vi "Get Selected Controls - List of properties.vi"(8 "error in (no error)":errorcluster, 10 "List of Properties":string[](array[string]), 11 "Data in":T2) -> (0 "error out":errorcluster, 3 "Selected Ctrls - List of Properties":T1)   [LabVIEW 2021, in "Control Property Tree.lvlib"]
uses:
  Control Property Tree.lvlib
  Module Data--cluster.ctl
  Ctrl Properties Map Data.ctl
  Property array.ctl
  Selected Ctrls - List of Controls.ctl
  Selected Ctrls - List of Properties.ctl
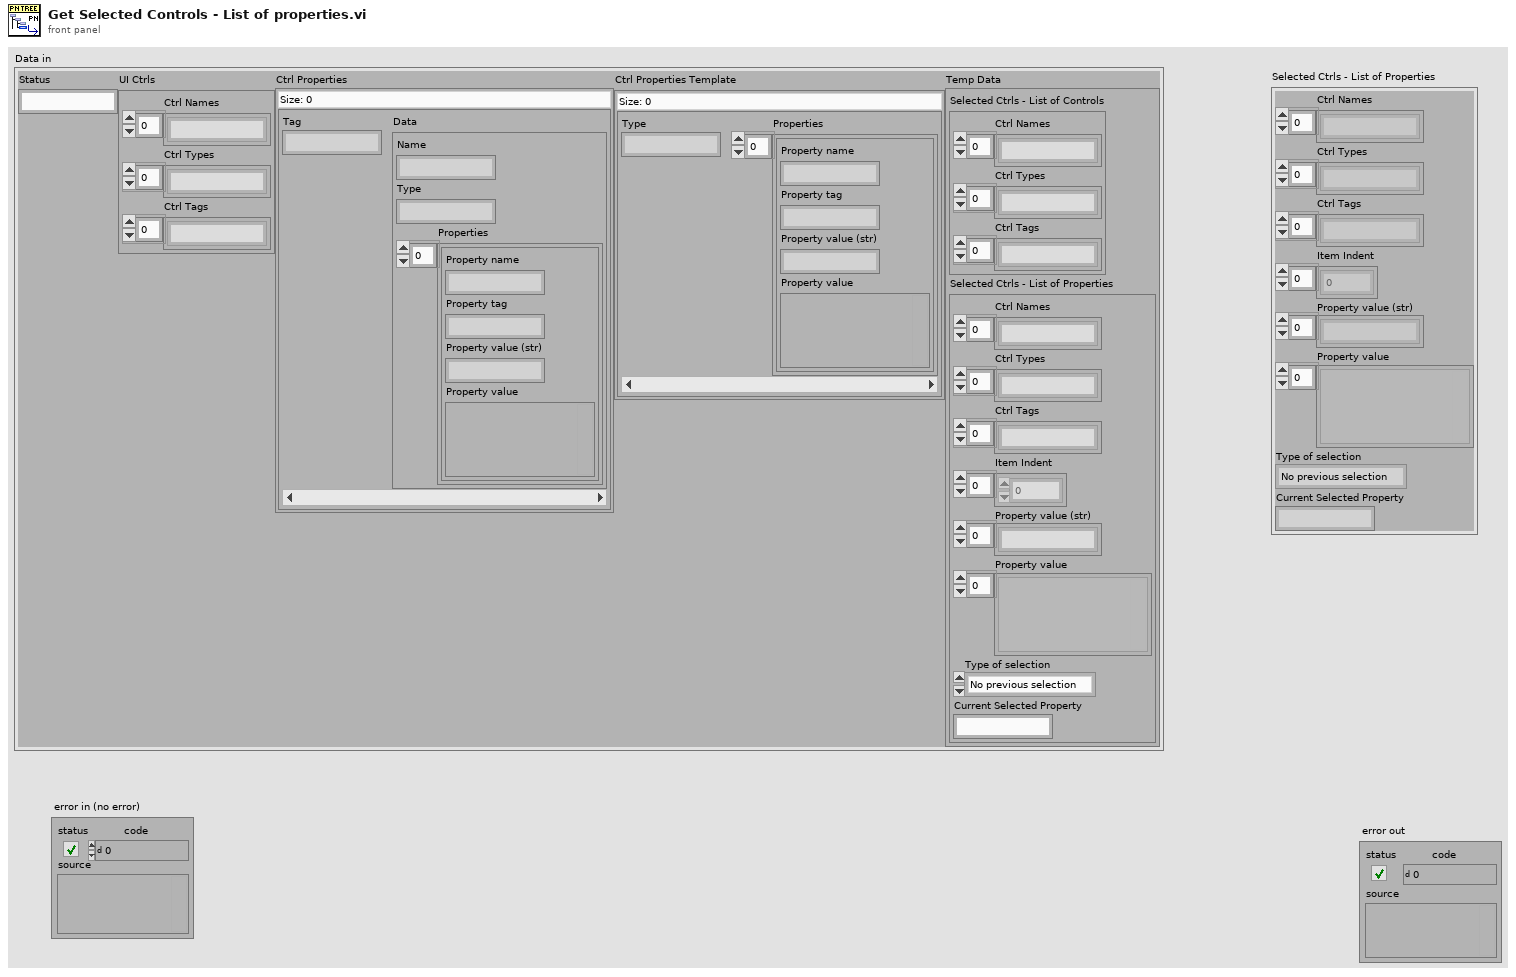
[diagram p1: front panel]
types:
  T1 = typedef "Control Property Tree.lvlib/Selected Ctrls - List of Properties.ctl" = cluster{"Ctrl Names":string[], "Ctrl Types":string[], "Ctrl Tags":string[], "Item Indent":i32[], "Property value (str)":string[], "Property value":variant[], "Type of selection":enum16{"No previous selection", "Control selected", "Property selected"}, "Current Selected Property":string}
  T2 = typedef "Control Property Tree.lvlib/Module Data--cluster.ctl" = cluster{"Status":string, "UI Ctrls":cluster{"Ctrl Names":string[], "Ctrl Types":string[], "Ctrl Tags":string[]}, "Ctrl Properties":map{string, T3}, "Ctrl Properties Template":map{string, T4}, "Temp Data":cluster{"Selected Ctrls - List of Controls":T5, "Selected Ctrls - List of Properties":T1}}
  T3 = typedef "Control Property Tree.lvlib/Ctrl Properties Map Data.ctl" = cluster{"Name":string, "Type":string, "Properties":T4}
  T4 = typedef "Control Property Tree.lvlib/Property array.ctl" = cluster{"Property name":string, "Property tag":string, "Property value (str)":string, "Property value":variant}[]
  T5 = typedef "Control Property Tree.lvlib/Selected Ctrls - List of Controls.ctl" = cluster{"Ctrl Names":string[], "Ctrl Types":string[], "Ctrl Tags":string[]}
  T6 = enum16{"No previous selection", "Control selected", "Property selected"}
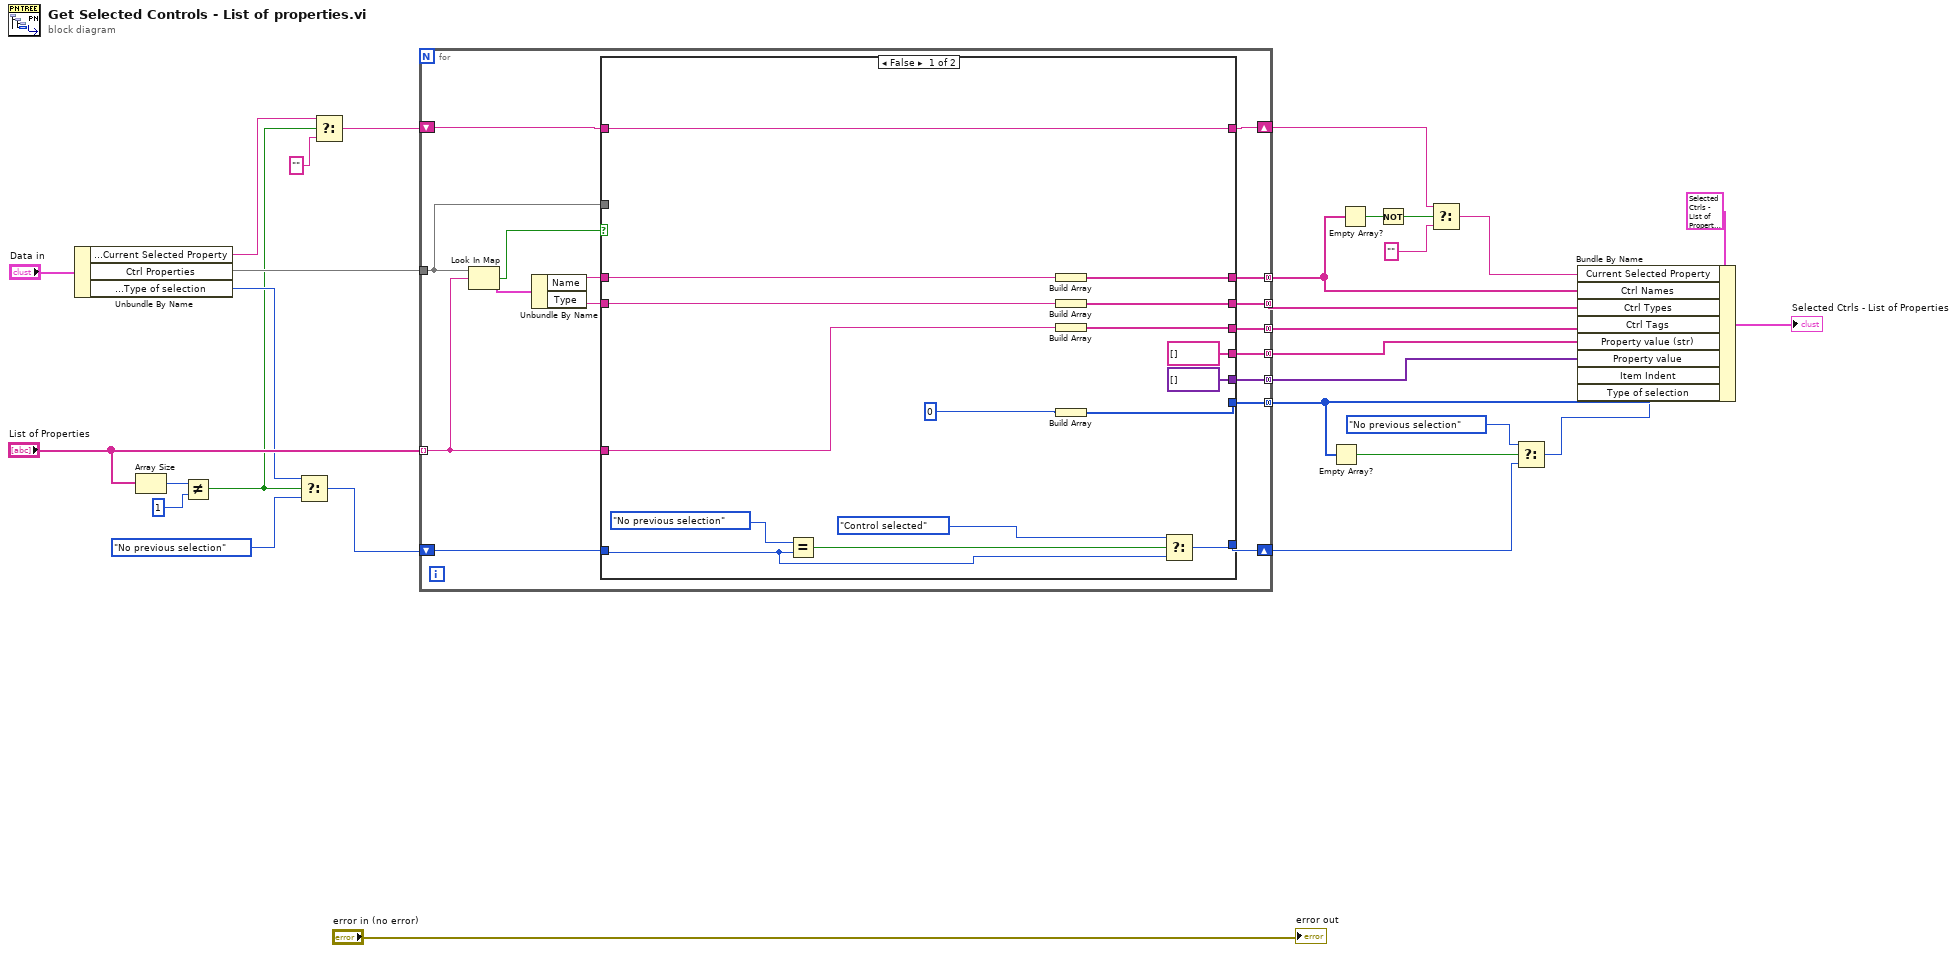
[diagram p0: block diagram]
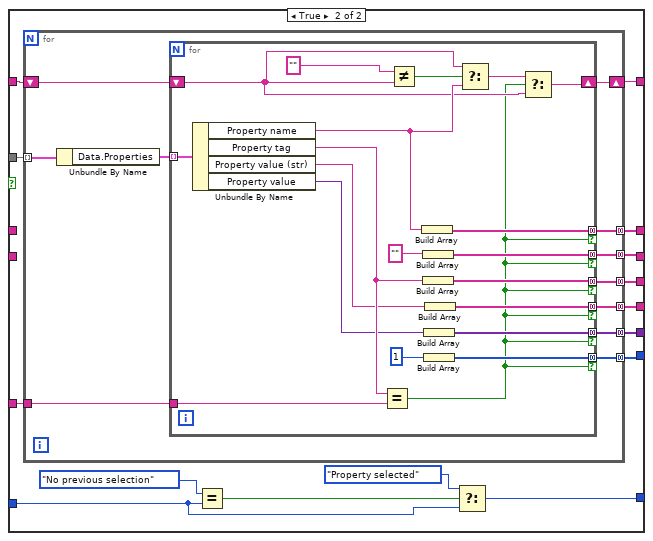
[diagram p2: hidden frame]
diagram:
  n1 = Unbundle By Name("Data in") -> ("Temp Data.Selected Ctrls - List of Properties.Current Selected Property"=w6:string, "Ctrl Properties"=w28:map{string, T3}, "Temp Data.Selected Ctrls - List of Properties.Type of selection"=w16:T6)
  n2 = Array Size(array="List of Properties") -> (size(s)=w18:i32)
  n3 = Not Equal?(x=w18, y=1) -> (x != y?=w3:bool)
  n4 = Select(t=w16, s=w3, f=T6."No previous selection") -> (s? t:f=w14:T6)
  n5 = Select(t=w6, s=w3, f="") -> (s? t:f=w5:string)
  n6 = for {
    tunnel: w28 -> [w45]
    tunnel: "List of Properties" -> [w42] mode=indexing
    tunnel: [w39] -> w12 mode=concatenating
    tunnel: [w41] -> w25 mode=concatenating
    tunnel: [w43] -> w24 mode=concatenating
    tunnel: [w37] -> w23 mode=concatenating
    shift-right: [w35] -> w21
    shift-left: w14 -> [w36]
    shift-right: [w33] -> w9
    shift-left: w5 -> [w34]
    tunnel: [w32] -> w2 mode=concatenating
    tunnel: [w31] -> w1 mode=concatenating
    n7 = Look In Map(map=w45, key=w42) -> (key not found?=w44:bool, value=w46:T3)  [unwired: 1 in]
    n8 = Unbundle By Name(w46) -> ("Name"=w38:string, "Type"=w40:string)
    n9 = case shown="False" w44 {
      tunnel: w45 -> [_ w77]
      tunnel: [w59 w74] -> w43
      tunnel: w42 -> [w58 w76]
      tunnel: [w61 w72] -> w41
      tunnel: w40 -> [w60 _]
      tunnel: [w62 w73] -> w39
      tunnel: w38 -> [w50 _]
      tunnel: [w56 w75] -> w37
      tunnel: w36 -> [w53 w70]
      tunnel: [w54 w69] -> w35
      tunnel: w34 -> [w49 w66]
      tunnel: [w49 w65] -> w33
      tunnel: [string[] [] w64] -> w32
      tunnel: [variant[] [] w63] -> w31
      frame False {
        n10 = Equal?(x=T6."No previous selection" ("Temp Data.Selected Ctrls - List of Properties.Type of selection"), y=w53) -> (x = y?=w55:bool)
        n11 = Build Array(w50) -> (w62:string[])
        n12 = Build Array(w60) -> (w61:string[])
        n13 = Build Array(w58) -> (w59:string[])
        n14 = Build Array(0) -> (w56:i32[])
        n15 = Select(t=T6."Control selected" ("Temp Data.Selected Ctrls - List of Properties.Type of selection"), s=w55, f=w53) -> (s? t:f=w54:T6)
      }
      frame True {
        n16 = for {
          tunnel: w77 -> [w88] mode=indexing
          tunnel: w76 -> [w86]
          tunnel: [w85] -> w75 mode=concatenating
          tunnel: [w84] -> w74 mode=concatenating
          tunnel: [w83] -> w73 mode=concatenating
          tunnel: [w82] -> w72 mode=concatenating
          shift-right: [w80] -> w65
          shift-left: w66 -> [w81]
          tunnel: [w79] -> w64 mode=concatenating
          tunnel: [w78] -> w63 mode=concatenating
          n17 = Unbundle By Name(w88) -> ("Data.Properties"=w87:T4)
          n18 = for {
            tunnel: w87 -> [w108] mode=indexing
            tunnel: w86 -> [w107]
            tunnel: [w100] -> w85 mode=concatenating if=w89
            tunnel: [w105] -> w84 mode=concatenating if=w89
            tunnel: [w106] -> w83 mode=concatenating if=w89
            tunnel: [w102] -> w82 mode=concatenating if=w89
            shift-right: [w94] -> w80
            shift-left: w81 -> [w95]
            tunnel: [w92] -> w79 mode=concatenating if=w89
            tunnel: [w90] -> w78 mode=concatenating if=w89
            n19 = Unbundle By Name(w108) -> ("Property name"=w98:string, "Property tag"=w104:string, "Property value (str)"=w93:string, "Property value"=w91:variant)
            n20 = Equal?(x=w104, y=w107) -> (x = y?=w89:bool)
            n21 = Not Equal?(x="", y=w95) -> (x != y?=w97:bool)
            n22 = Build Array(w98) -> (w106:string[])
            n23 = Build Array("") -> (w102:string[])
            n24 = Build Array(w104) -> (w105:string[])
            n25 = Build Array(w91) -> (w90:variant[])
            n26 = Build Array(1) -> (w100:i32[])
            n27 = Build Array(w93) -> (w92:string[])
            n28 = Select(t=w95, s=w97, f=w98) -> (s? t:f=w96:string)
            n29 = Select(t=w96, s=w89, f=w95) -> (s? t:f=w94:string)
          }
        }
        n30 = Equal?(x=T6."No previous selection" ("Temp Data.Selected Ctrls - List of Properties.Type of selection"), y=w70) -> (x = y?=w71:bool)
        n31 = Select(t=T6."Property selected" ("Temp Data.Selected Ctrls - List of Properties.Type of selection"), s=w71, f=w70) -> (s? t:f=w69:T6)
      }
    }
  }
  n32 = Empty Array?(array=w23) -> (empty?=w22:bool)
  n33 = Empty Array?(array=w12) -> (empty?=w11:bool)
  n34 = Not(x=w11) -> (.not. x?=w10:bool)
  n35 = Select(t=w9, s=w10, f="" ("x")) -> (s? t:f=w7:string)
  n36 = Select(t=T6."No previous selection" ("f"), s=w22, f=w21) -> (s? t:f=w20:T6)
  n37 = Bundle By Name(cluster=T1 {"Ctrl Names"=[], "Ctrl Types"=[], "Ctrl Tags"=[], "Item Indent"=[], "Property value (str)"=[], "Property value"=[], "Type of selection"=enum."No previous selection", "Current Selected Property"=""} ("Selected Ctrls - List of Properties"), "Current Selected Property"=w7, "Ctrl Names"=w12, "Ctrl Types"=w25, "Ctrl Tags"=w24, "Property value (str)"=w2, "Property value"=w1, "Item Indent"=w23, "Type of selection"=w20) -> (→"Selected Ctrls - List of Properties":T1)
  "error out" <- "error in (no error)"
